vi "4134 Process Controls.vi"(8 "Remote 2 Packet":string, 9 "Remote 1 Packet":string, 10 "Enabled? (Default)":enum16{"Disabled", "Enabled"}(ring)=enum."Enabled", 11 "NXT":T3={"Hardware"="NXT", "Flattened String"=""}) -> (0 "Controller 2 State":T1={"Left X"=0, "Left Y"=0, "Right X"=0, "Right Y"=0, "Button Encoding 9-12"=0, "Button Encoding 1-8"=0, "POV"=-1} {"POV" items=["None"=-1, "POV Up"=0, "POV Up Right"=1, "POV Right"=2, "POV Down Right"=3, "POV Down"=4, "POV Down Left"=5, "POV Left"=6, "POV Up Left"=7]}, 1 "Controller 1 State":T1={"Left X"=0, "Left Y"=0, "Right X"=0, "Right Y"=0, "Button Encoding 9-12"=0, "Button Encoding 1-8"=0, "POV"=-1} {"POV" items=["None"=-1, "POV Up"=0, "POV Up Right"=1, "POV Right"=2, "POV Down Right"=3, "POV Down"=4, "POV Down Left"=5, "POV Left"=6, "POV Up Left"=7]}, 3 "NXT":T3={"Hardware"="NXT", "Flattened String"=""})   [LabVIEW 2010, in "FTC.lvlib" / "Remote Interface.lvlib"]
uses:
  Remote Interface.lvlib
  <vilib>/NXT/Subs/LVHSConnector.ctl
  <vilib>/FTC/FTC ControllerState.ctl
  <vilib>/FTC/FTC POVState.ctl
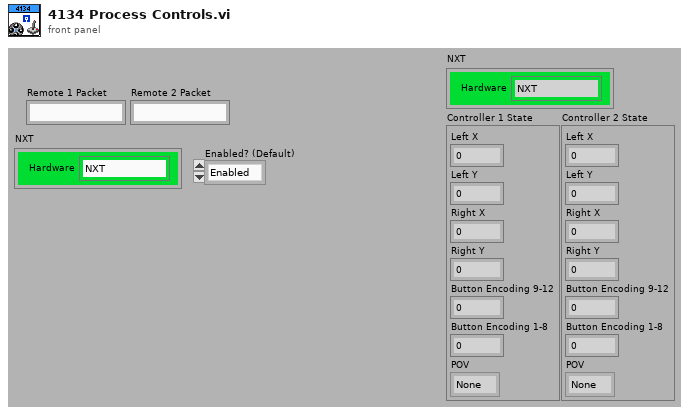
[diagram p1: front panel]
types:
  T1 = typedef "FTC ControllerState.ctl" = cluster{"Left X":i8, "Left Y":i8, "Right X":i8, "Right Y":i8, "Button Encoding 9-12":u8, "Button Encoding 1-8":u8, "POV":T2}
  T2 = typedef "FTC POVState.ctl" = i8
  T3 = typedef "LVHSConnector.ctl" = cluster{"Hardware":string, "Flattened String":string}
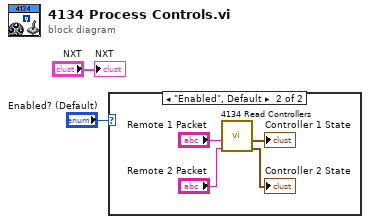
[diagram p0: block diagram]
diagram:
  n1 = case shown="\"Enabled\", Default" "Enabled? (Default)" {
    frame "Disabled" {
    }
    frame "Enabled", Default {
      n2 = call "4134 Read Controllers.vi"("Remote 2 Packet"="Remote 2 Packet", "Remote 1 Packet"="Remote 1 Packet") -> ("Controller 2 State"=→"Controller 2 State":T1, "Controller 1 State"=→"Controller 1 State":T1)  [unwired: 7 in, 1 out]
    }
  }
  "NXT" <- "NXT"
